vi "T6.vi"() -> ()   [LabVIEW 2020]
panel:
  out "A este egal cu B":bool
  out "A este mai mic ca B":bool
  out "A este mai mare ca B":bool
  in  "B":dbl
  in  "A":dbl
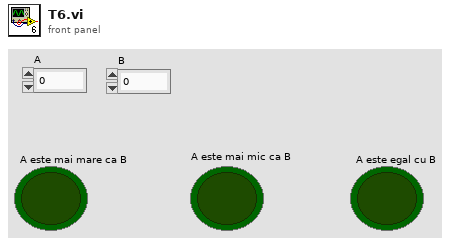
[diagram p1: front panel]
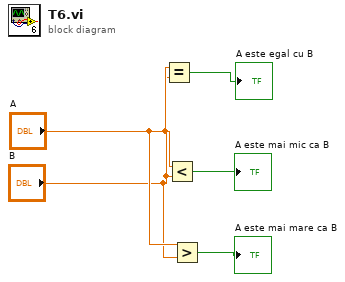
[diagram p0: block diagram]
diagram:
  n1 = Equal?(x="A", y="B") -> (x = y?=→"A este egal cu B":bool)
  n2 = Less?(x="A", y="B") -> (x < y?=→"A este mai mic ca B":bool)
  n3 = Greater?(x="A", y="B") -> (0:→"A este mai mare ca B":bool)
